vi "editDialog.vi"(0 "reference":refnum<class "StateDiagramGraph.lvclass">, 5 "error in (no error)":errorcluster) -> (14 "reference out":refnum<class "StateDiagramGraph.lvclass">, 16 "cancel":bool, 19 "error out":errorcluster)   [LabVIEW 2016, in "StateDiagramGraph.lvclass"]
doc: "Edit Dialog"
uses:
  <resource>/Framework/Providers/Open_GDS/UML/StateDiagramGraph_class/StateDiagramGraph.lvclass
  <resource>/Framework/Providers/Open_GDS/UML/StateDiagramGraph_class/private/ViPathShowOption.ctl
  <resource>/Framework/Providers/Open_GDS/UML/ContextHelp/ContextHelp_HelpTexts.ctl
panel:
  in  "VI-Name Show Option":T1
  in  "OK Button":bool
  in  "Cancel Button":bool
  in  "Help":bool
  in  "VI-Path":path
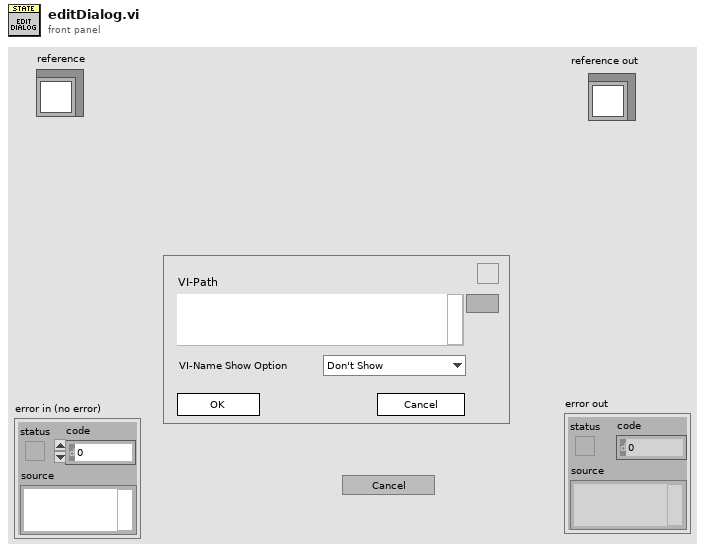
[diagram p1: front panel]
types:
  T1 = typedef "StateDiagramGraph.lvclass/ViPathShowOption.ctl" = enum16{"Don't Show", "Show Relative Path", "Show Absolute Path"}
  T2 = typedef "ContextHelp_HelpTexts.ctl" = enum16{"None(Hide)", "Default", "Help", "Welcome", "GettingStarted", "ClassDiagram_Help", "SequenceDiagram_Help", "UseCaseDiagram_Help", "BSelect", "BClass", "BInterface", "BPackage", "BNote", "BDependency", "BInheritance", "BInterfaceImplementation", "BAssociation", "BAggregation", "BCompAggregation", "BNoteConnector", "BObject", "BActionBar", "BCall", "BSystem", "BActor", "BUseCase", "BGeneralization", "BIncludes", "BExtends", "BUseCaseDiagramAssociation", "ClassRelationshipEdge editDialog_Bent Style", "ClassRelationshipEdge editDialog_RelationType", "ClassRelationshipEdge editDialog_Reverse association", "ClassRelationshipEdge editDialog_Start label", "ClassRelationshipEdge editDialog_Middle label", "ClassRelationshipEdge editDialog_End label", "UMLEditor reversedEngineering_Pathes", "ReversedEngineering StateReverseDialog_Help", "ReversedEngineering StateQueuedSettings_Help", "UMLEditor reversedEngineering_AddTopVIs", "UMLEditor reversedEngineering_AddClasses", "UMLEditor reversedEngineering_AddDirs", "UMLEditor reversedEngineering_Recursively", "UMLEditor reversedEngineering_Remove", "UMLEditor reversedEngineering_ClearList", "UMLEditor reversedEngineering_HideSubAss", "UMLEditor reversedEngineering_CreateTypes", "UMLEditor reversedEngineering_OnlyInheritance", "UMLEditor reversedEngineering_CreateApplication", "UMLEditor reversedEngineering_OK", "UMLEditor reversedEngineering_Cancel", "UMLEditor reversedEngineering_Help", "UMLEditor createWizardScriptFile_ScriptfilePath", "UMLEditor createWizardScriptFile_ClassPath", "UMLEditor createWizardScriptFile_Use", "UMLEditor createWizardScriptFile_PrivateDirName", "UMLEditor createWizardScriptFile_DirAppend", "UMLEditor createWizardScriptFile_Separator Character", "UMLEditor createWizardScriptFile_OK", "UMLEditor createWizardScriptFile_Cancel", "UMLEditor createWizardScriptFile_Help", "ClassNode editDialog_Class Name", "InterfaceNode editDialog_Class Name", "ClassNode editDialog_Attribute", "ClassNode editDialog_Methods", "InterfaceNode editDialog_Methods", "ClassNode editDialog_connection", "InterfaceNode editDialog_connection", "ClassNode editDialog_StereoType", "ClassNode editDialog_ShowAttrib", "ClassNode editDialog_ShowMethods", "ClassNode editDialog_ClassPath", "ClassNode editDialog_AddAttribute", "ClassNode editDialog_AddMethod", "InterfaceNode editDialog_AddMethod", "ClassNode AttributeGuide_AttributeName", "ClassNode AttributeGuide_Array?", "ClassNode AttributeGuide_Data Type", "ClassNode AttributeGuide_RefName", "ClassNode AttributeGuide_Preview", "ClassNode AttributeGuide_OK", "ClassNode AttributeGuide_Cancel", "ClassNode MethodGuide_Visibility", "ClassNode MethodGuide_Method Name", "ClassNode MethodGuide_Preview", "ClassNode MethodGuide_OK", "ClassNode MethodGuide_Cancel", "CallNode EditCallProperties_AllButtons", "ObjectNode EditObjectlProperties_AllButtons", "ActorNode EditActorProperties_AllButtons", "UseCaseRelationshipNode EditUseCaselProperties_AllButtons", "UseCaseNode EditUseCaselProperties_AllButtons", "SystemNode EditSystemProperties_AllButtons", "ReversedEngineering UpdateAttributes_AllButtons", "StateNode editDialog_AllButtons", "StateTransition editDialog_AllButtons", "ArrangeNodes Main_Picture", "ArrangeNodes Main_Zoom", "ArrangeNodes Main_Auto Zoom", "ArrangeNodes Main_shorten", "ArrangeNodes Main_Min Length", "ArrangeNodes Main_Max Length", "ArrangeNodes Main_increase", "ArrangeNodes Main_decrease", "ArrangeNodes Main_Shake", "ArrangeNodes Main", "BState", "BInitialState", "BFinalState", "BStateTransition", "StateDiagram_Help", "StateDiagram_PropertiesAllButtons", "ReversedEngineering StateReverseDialog_ClearStates", "ReversedEngineering StateReverseDialog_UseQueuedStateMachines", "ReversedEngineering StateReverseDialog_QueuedSettings", "ReversedEngineering StateReverseDialog_SearchForVIs", "ReversedEngineering StateReverseDialog_SearchCriteria", "OptionsDialog_ClassBasePath", "OptionsDialog_VIPath", "OptionsDialog_ApplicationPath", "OptionsDialog_WizDir", "OptionsDialog_IniFilePath", "OptionsDialog_DefineColors", "OptionsDialog_Help", "OptionsDialog_CreateTypes", "ClassRelationshipEdge editDialog_SplitWire"}
  T3 = typedef "StateDiagramGraph.lvclass/ObjectAttributes.ctl" = cluster{"StateDiagramData":T4}
  T4 = typedef "StateDiagramGraph.lvclass/StateDiagramData.ctl" = cluster{"VI-Path":path, "ShowOption":T1}
  T5 = typedef "ContextHelp_ShowType.ctl" = cluster{"Header":string, "Picture":picture, "Text":string}
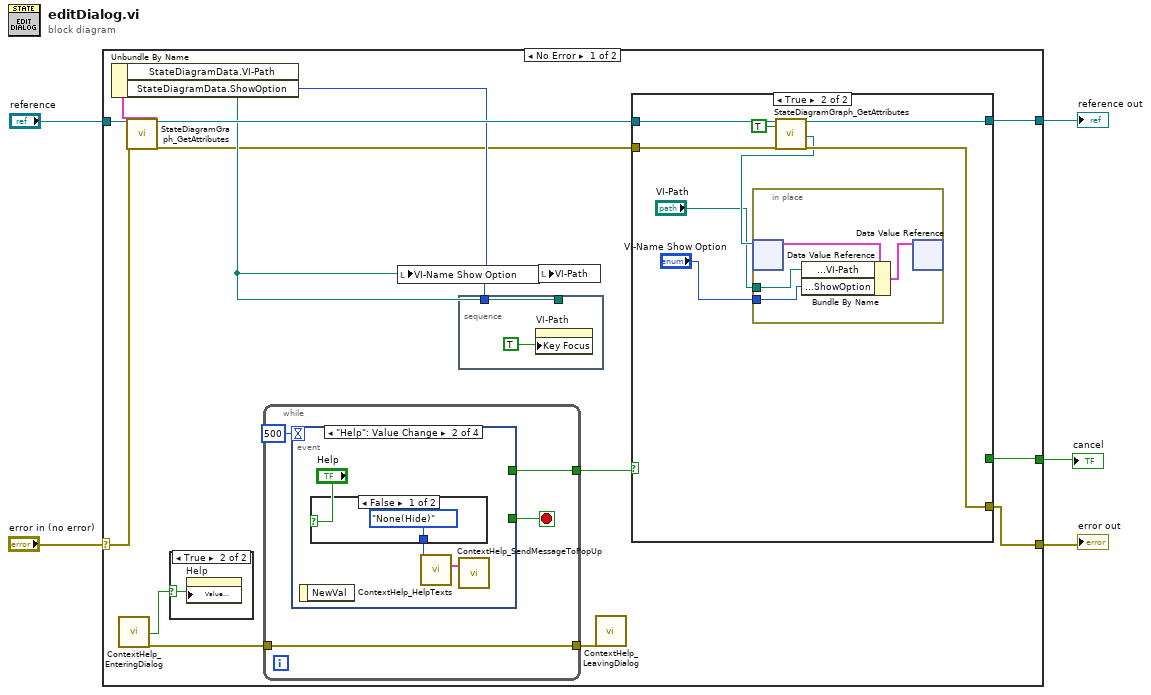
[diagram p0: block diagram]
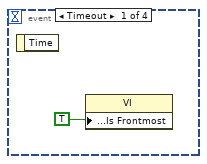
[diagram p3: hidden frame]
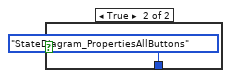
[diagram p4: hidden frame]
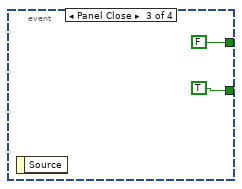
[diagram p5: hidden frame]
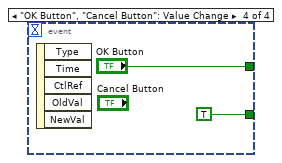
[diagram p6: hidden frame]
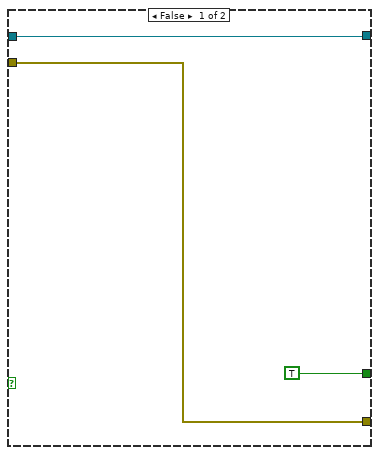
[diagram p7: hidden frame]
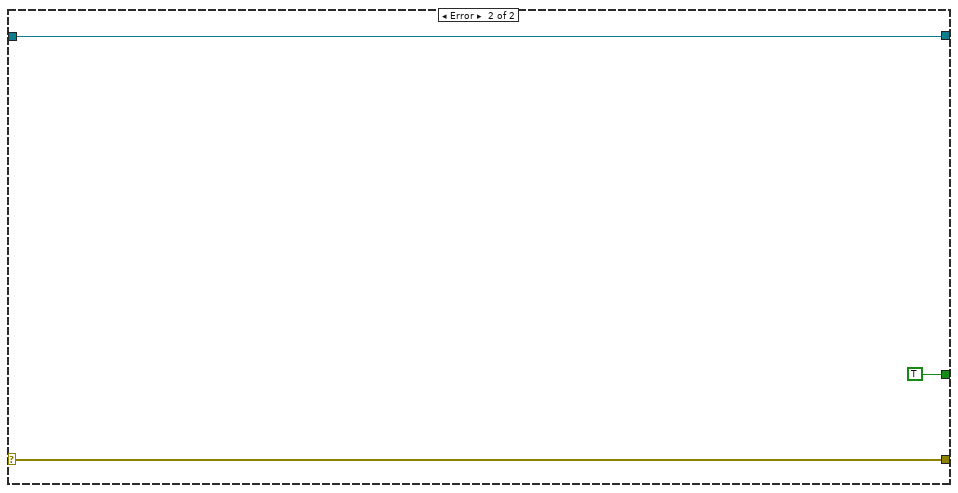
[diagram p8: hidden frame]
diagram:
  n1 = case shown="No Error" "error in (no error)" {
    selector: "error in (no error)" -> [w15 w52]
    tunnel: "reference" -> [w16 w53]
    tunnel: [w19 w52] -> w3
    tunnel: [w18 w53] -> w2
    tunnel: [w14 TRUE ("Key Focus")] -> w1
    frame No Error {
      n2 = call <resource>:"ContextHelp_EnteringDialog.vi"() -> ("HelpStatus"=w10:bool, "error out"=w12:errorcluster)  [unwired: 3 in, 15 out]
      n3 = call <resource>:"StateDiagramGraph_GetAttributes.vi"("reference in"=w16, "error in (no error)"=w15) -> ("reference out"=w17:refnum<class "StateDiagramGraph.lvclass">, "Data"=w6:T3, "error out"=w7:errorcluster)  [unwired: 1 in, 14 out]
      n4 = Unbundle By Name(w6) -> ("StateDiagramData.VI-Path"=w9:path, "StateDiagramData.ShowOption"=w8:T1)
      n5 = case shown="True" w10 {
        selector: w10 -> [_ w20]
        frame False {
        }
        frame True {
          n6 = property on="Help" class="Bool (strict)"("Value (Signaling)"=w20) -> ()  [unwired: 2 in, 2 out]
        }
      }
      n7 = while {
        tunnel: [w24] -> w11
        tunnel: [w22] -> w13
        tunnel: w12 -> [w22]
        stop <- w23 stop-if-true
        n8 = event shown="[1] \"Help\": Value Change" {
          selector: _ -> [_ _ _ _]
          dyn-events: _ -> [_ _ _ _]
          timeout: 500 -> [_ _ _ _]
          tunnel: [_ _ FALSE ("OK Button") "OK Button"] -> w24
          tunnel: [_ _ TRUE ("OK Button") TRUE] -> w23
          event Timeout {
            n9 = event-data() -> ()  [unwired: 2 out]
            n10 = property class="VI"("Front Panel Window:Is Frontmost"=TRUE) -> ()  [unwired: 2 in, 2 out]
          }
          event "Help": Value Change {
            n11 = event-data() -> ()  [unwired: 2 out]
            n12 = case shown="False" "Help" {
              tunnel: [ContextHelp_HelpTexts."None(Hide)" ("HelpText") ContextHelp_HelpTexts."StateDiagram_PropertiesAllButtons" ("HelpText")] -> w27
              frame False {
              }
              frame True {
              }
            }
            n13 = call <resource>:"ContextHelp_HelpTexts.vi"("HelpText (enum or string)"=w27) -> ("HelpOut"=w28:T5)  [unwired: 18 out]
            n14 = call <resource>:"ContextHelp_SendMessageToPopUp.vi"("PopUpMessage"=w28) -> ()  [unwired: 2 in, 17 out]
          }
          event Panel Close {
            n15 = event-data() -> ()  [unwired: 2 out]
          }
          event "OK Button", "Cancel Button": Value Change {
            n16 = event-data() -> ()  [unwired: 6 out]
          }
        }
      }
      n17 = local write "VI-Name Show Option"(w8) -> ()
      n18 = stacked-sequence {
        tunnel: w9 -> [_]
        tunnel: w8 -> [_]
        frame #0 {
          n19 = property on="VI-Path" class="Path"("Key Focus"=TRUE) -> ()  [unwired: 2 in, 2 out]
        }
      }
      n20 = local write "VI-Path"(w9) -> ()
      n21 = call <resource>:"ContextHelp_LeavingDialog.vi"("error in (no error)"=w13) -> ()  [unwired: 2 in, 17 out]
      n22 = case shown="True" w11 {
        tunnel: [w36 w42] -> w19
        tunnel: [w37 w44] -> w18
        tunnel: w17 -> [w37 w45]
        tunnel: w7 -> [w36 w43]
        tunnel: [TRUE ("Key Focus") _] -> w14
        frame False {
        }
        frame True {
          n23 = call <resource>:"StateDiagramGraph_GetAttributes.vi"("reference in"=w45, "OnlyGetDvrReference(False)"=TRUE, "error in (no error)"=w43) -> ("reference out"=w44:refnum<class "StateDiagramGraph.lvclass">, "DataRef"=w40:refnum<data-value>, "error out"=w42:errorcluster)  [unwired: 13 in, 1 out]
          n24 = in-place {
            in-place-border: "VI-Path" -> [w48]
            in-place-border: "VI-Name Show Option" -> [w47]
            n25 = in-place-dvr #1(w40) -> (w49:T3)  [unwired: 1 out]
            n26 = Bundle By Name(cluster=w49, "StateDiagramData.VI-Path"=w48, "StateDiagramData.ShowOption"=w47) -> (w46:T3)
            n27 = in-place-dvr #1(w46) -> ()  [unwired: 2 out]
          }
        }
      }
    }
    frame Error {
    }
  }
  "reference out" <- w2
  "error out" <- w3
  "cancel" <- w1
